vi "byte20-23 (SubVI).vi"(11 "unsigned byte array":u8[](array[numeric])) -> (2 "Numeric":u16, 3 "Numeric 2":u16)   [LabVIEW 2016]
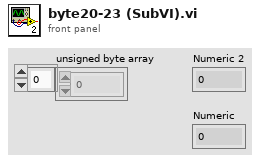
[diagram p1: front panel]
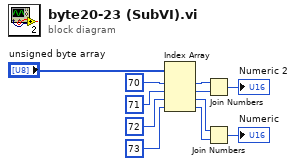
[diagram p0: block diagram]
diagram:
  n1 = Index Array(array="unsigned byte array", index #1=70 ("index"), index #2=71 ("index"), index #3=72 ("index"), index #4=73 ("index")) -> (element #1=w5:u8, element #2=w6:u8, element #3=w7:u8, element #4=w8:u8)
  n2 = Join Numbers(hi=w5, lo=w6) -> ((hi.lo)=→"Numeric 2":u16)
  n3 = Join Numbers(hi=w7, lo=w8) -> ((hi.lo)=→"Numeric":u16)
